vi "Launch Wind Turbine.vi"(6 "File Type":T1, 8 "error in":errorcluster, 9 "Front Panel Open?":bool, 10 "Calling VI Path":path, 11 "VIT Path":path) -> (0 "error out":errorcluster, 2 "Name":string, 3 "vi reference":refnum<vi>)   [LabVIEW 2009]
doc: "This is the launcher for the Wind Turbines which are created from a .vit.\n\nAAL 9/09"
uses:
  Controls/File Type.ctl
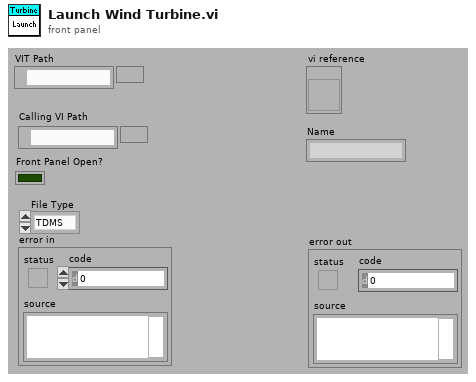
[diagram p1: front panel]
types:
  T1 = typedef "File Type.ctl" = enum16{"TDMS", "TXT"}
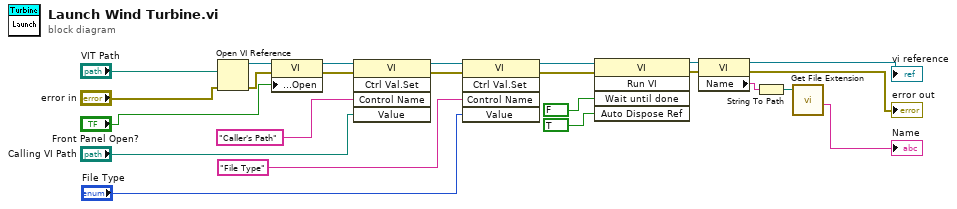
[diagram p0: block diagram]
diagram:
  n1 = Open VI Reference(vi path="VIT Path", error in (no error)="error in") -> (vi reference=w17:refnum<vi>, error out=w18:errorcluster)  [unwired: 4 out]
  n2 = property class="VI"(reference=w17, error in=w18, "Front Panel.Open"="Front Panel Open?") -> (reference out=w14:refnum<vi>, error out=w13:errorcluster)
  n3 = invoke class="VI" method="Ctrl Val.Set"(reference=w14, error in=w13, "Control Name"="Caller's Path", "Value"="Calling VI Path") -> (reference out=w6:refnum<vi>, error out=w5:errorcluster)  [unwired: 1 in, 3 out]
  n4 = invoke class="VI" method="Ctrl Val.Set"(reference=w6, error in=w5, "Control Name"="File Type", "Value"="File Type") -> (reference out=w4:refnum<vi>, error out=w3:errorcluster)  [unwired: 1 in, 3 out]
  n5 = invoke class="VI" method="Run VI"(reference=w4, error in=w3, "Wait until done"=FALSE ("Wait Until Done"), "Auto Dispose Ref"=TRUE ("Auto Dispose Reference")) -> (reference out=w23:refnum<vi>, error out=w16:errorcluster)  [unwired: 1 in, 3 out]
  n6 = property class="VI"(reference=w23, error in=w16) -> (reference out=→"vi reference":refnum<vi>, error out=→"error out":errorcluster, "Name"=w10:string)
  n7 = String To Path(string=w10) -> (path=w9:path)
  n8 = call <vilib>:"Get File Extension.vi"("file"=w9) -> ("filename without extension"=→"Name":string)  [unwired: 7 in, 3 out]
